vi "Check Labels Savable.vi"(8 "error in":errorcluster, 11 "Element Labels":string[](array[string])) -> (0 "error out":errorcluster)   [LabVIEW 2023, in "Label-Driven UI.lvlib"]
uses:
  Label-Driven UI.lvlib
  <vilib>/ErrorRing/Error Ring.xnode
  <vilib>/Utility/error.llb/Error Cluster From Error Code.vi
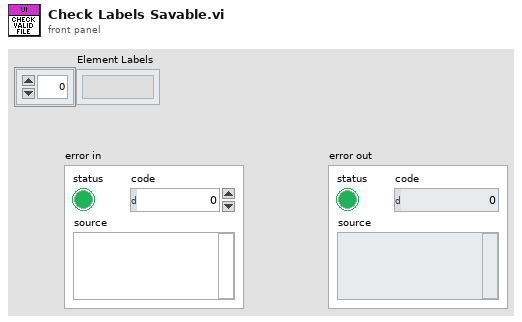
[diagram p1: front panel]
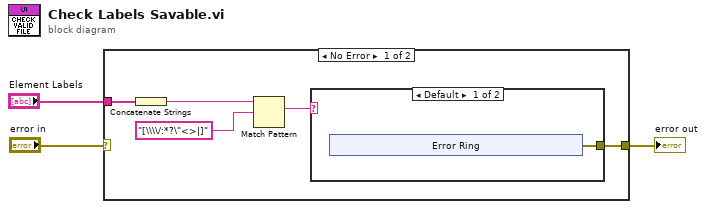
[diagram p0: block diagram]
diagram:
  n1 = case shown="No Error" "error in" {
    selector: "error in" -> [_ w15]
    tunnel: [w4 w15] -> w2
    tunnel: "Element Labels" -> [w8 _]
    frame No Error {
      n2 = Concatenate Strings(w8) -> (w7:string)
      n3 = Match Pattern(string=w7, regular expression="[\\\\/:*?\"<>|]") -> (match substring=w5:string)  [unwired: 1 in, 3 out]
      n4 = case shown="Default" w5 {
        tunnel: [w9 _] -> w4
        frame Default {
          n5 = xnode "Error Ring"() -> ("error out"=w9:errorcluster)
        }
        frame "" {
        }
      }
    }
    frame Error {
    }
  }
  "error out" <- w2
